vi "Find Next Available Channel.vi"(9 "Starting Index (0)":i32, 11 "Channels Info":T1[](array[typedef])) -> (1 "Available Channel Index":i32, 3 "Next Channel Info":T1)   [LabVIEW 2021, in "myRIO Channel List.xctl"]
uses:
  <vilib>/myRIO/Common/Express VI Framework/xctls/myRIO Channel List/myRIO Channel List.xctl
  <vilib>/myRIO/Common/Profile Manager Framework/typedefs/Channel Info.ctl
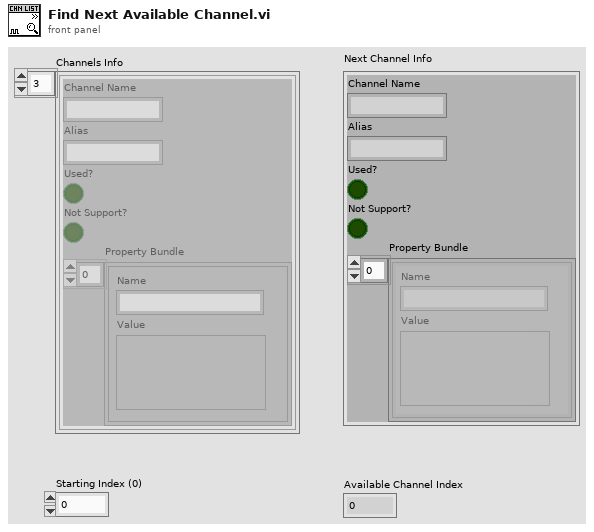
[diagram p1: front panel]
types:
  T1 = typedef "Channel Info.ctl" = cluster{"Channel Name":string, "Alias":string, "Used?":bool, "Not Support?":bool, "Property Bundle":cluster{"Name":string, "Value":variant}[]}
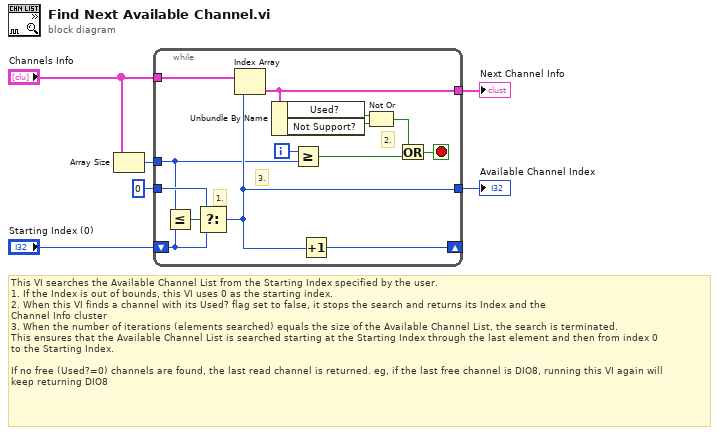
[diagram p0: block diagram]
diagram:
  # "This VI searches the Available Channel List from the Starting Index specified by the user. \n1. If the Index is out of bounds, this VI uses 0 as the starting index.\n2. When this VI finds a channel with its Used? flag set to false, it stops the search and returns its Index and the \nChannel Info cluster\n3. When the number of iterations (elements searched) equals the size of the Available Channel List, the search is terminated.\nThis ensures that the Available Channel List is searched starting at the Starting Index through the last element and then from index 0\nto the Starting Index. \n\nIf no free (Used?=0) channels are found, the last read channel is returned. eg, if the last free channel is DIO8, running this VI again will\nkeep returning DIO8"
  n1 = Array Size(array="Channels Info") -> (size(s)=w1:i32)
  n2 = while {
    shift-right: [w20] -> _
    shift-left: "Starting Index (0)" -> [w11]
    tunnel: "Channels Info" -> [w19]
    tunnel: [w17] -> w6
    tunnel: w1 -> [w10]
    tunnel: [w13] -> w5
    tunnel: 0 ("f") -> [w12]
    i -> [w18]
    stop <- w15 stop-if-true
    # "1."
    # "3."
    # "2."
    n3 = Less Or Equal?(x=w10, y=w11) -> (x <= y?=w14:bool)
    n4 = Select(t=w12, s=w14, f=w11) -> (s? t:f=w13:i32)
    n5 = Index Array(array=w19, index=w13) -> (element=w17:T1)
    n6 = Unbundle By Name(w17) -> ("Used?"=w9:bool, "Not Support?"=w8:bool)
    n7 = Greater Or Equal?(x=w18, y=w10) -> (x >= y?=w16:bool)
    n8 = Increment(x=w13) -> (x+1=w20:i32)
    n9 = Not Or(1:w8, 2:w9) -> (0:w7:bool)
    n10 = Or(x=w7, y=w16) -> (x .or. y?=w15:bool)
  }
  "Available Channel Index" <- w5
  "Next Channel Info" <- w6
